vi "source sim.vi"() -> ()   [LabVIEW 2016]
uses:
  <vilib>/Platform/TimedLoop/XDataNode/timing_clust.ctl
  <vilib>/Platform/TimedLoop/XDataNode/nitl_modes.ctl
  <vilib>/Platform/TimedLoop/XDataNode/wakeup.ctl
  <vilib>/Analysis/baseanly.llb/Mean (CDB).vi
  <vilib>/platform/TimedLoop/XDataNode/XDataNode.xnode
  <vilib>/Platform/TimedLoop/XDataNode/XDNodeRunTimeDep.lvlib
  <vilib>/Analysis/NI_AALBase.lvlib
panel:
  in  "Rotate CCW":bool
  in  "Rotate CW":bool
  in  "Stop Button":bool
  out "Simulation Time (Seconds)":dbl=0.12610000000000002 format="%_4g"
  out "Frequency (Hz)":dbl=34.3
  out "Wavenumber (Radians / Meter)":dbl=0.6283185307179586
  in  "Delete Source":bool
  in  "Add Source":bool
  in  "Velocity of Propogation (m/s)":dbl=343.0 min=200.0 max=400.0 step=1.0
  in  "dT":dbl=0.0001
  in  "Spatial Resolution (meters)":dbl=0.25 min=0.1 max=10.0 step=0.1
  in  "Extent (Meters)":dbl=50.0 min=50.0 max=400.0 step=1.0
  in  "Wavelength (meters)":dbl=10.0
  out "Intensity Graph":dbl[][](graph)
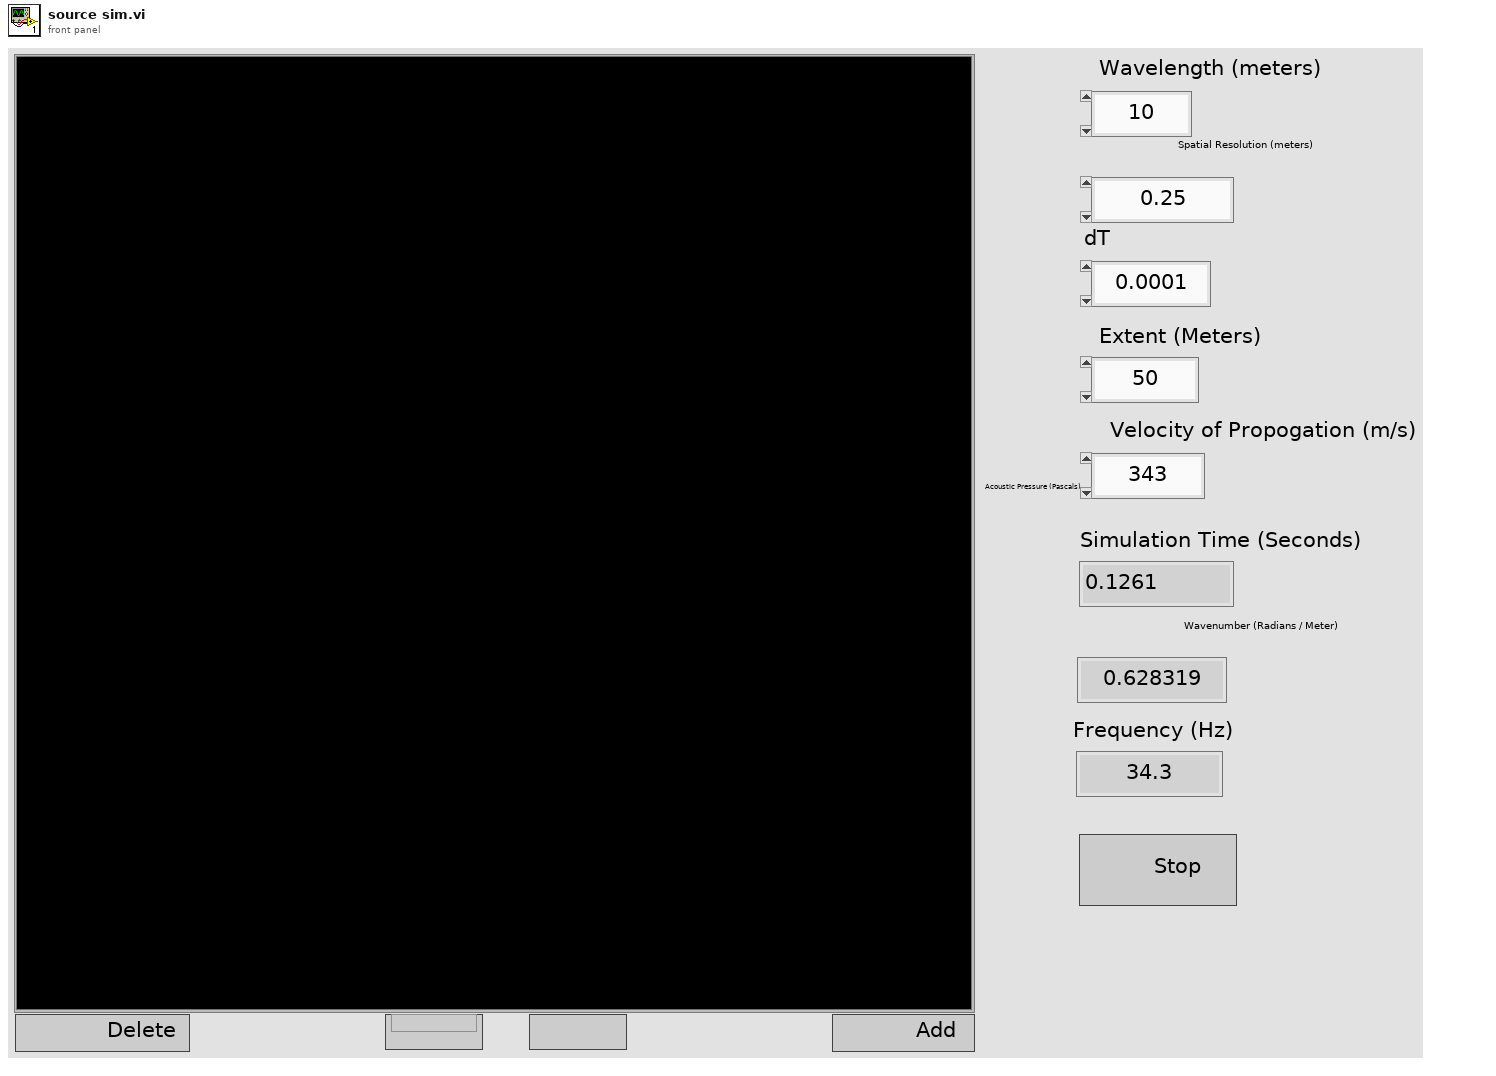
[diagram p1: front panel]
types:
  T1 = typedef "XDNodeRunTimeDep.lvlib/timing_clust.ctl" = cluster{"Expected End [f-1]":u64, "Actual End [f-1]":u64, "Finished Late? [f-1]":bool, "Expected End [i-1]":u64, "Actual End [i-1]":u64, "Finished Late? [i-1]":bool, "Expected Start [i]":u64, "Actual Start [i]":u64, "Expected Start [f]":u64, "Actual Start [f]":u64, "Source Name":string, "Structure Name":string, "Period":i64, "Deadline":i64, "Offset":i64, "Start":i64, "Priority":i32, "Timeout":i32, "Mode":T2, "Wakeup Reason":T3, "Error":errorcluster, "Source Type":string, "Secondary Source Type":string, "Global End Time":u64, "Global Start Time":u64, "Frame Duration":u64, "Iteration Duration":u64, "Assigned CPU":i32, "I/O Scan Engine Mode":u32}
  T2 = typedef "XDNodeRunTimeDep.lvlib/nitl_modes.ctl" = enum32{"No Change", "Process missed periods, maintain original phase", "Discard missed periods, maintain original phase", "Process missed periods, ignore original phase", "Discard missed periods, ignore original phase"}
  T3 = typedef "XDNodeRunTimeDep.lvlib/wakeup.ctl" = enum32{"Normal", "Aborted", "Asynchronous wakeup", "Timing source error", "Timed loop error", "Timeout"}
  T4 = cluster{"Name":string, "Color":u32, "Style":u8, "Point Style":u8, "Name Visible":bool, "Allow Drag":bool, "Cursor Mode":u32, "Plot":i32, "Index":i32, "Position":cluster{"X":dbl, "Y":dbl}, "X Scale":u32, "Y Scale":u32, "Watch Plots":i32[], "Watch All Plots":bool, "Plot Area":i32, "Label Offset":cluster{"X":dbl, "Y":dbl}}
  T5 = typedef "LVCursorListTypeDef.ctl" = cluster{"Name":string, "Color":u32, "Style":u8, "Point Style":u8, "Name Visible":bool, "Allow Drag":bool, "Cursor Mode":u32, "Plot":i32, "Index":i32, "Position":cluster{"X":dbl, "Y":dbl}, "X Scale":u32, "Y Scale":u32, "Watch Plots":i32[], "Watch All Plots":bool, "Plot Area":i32, "Label Offset":cluster{"X":dbl, "Y":dbl}}[]
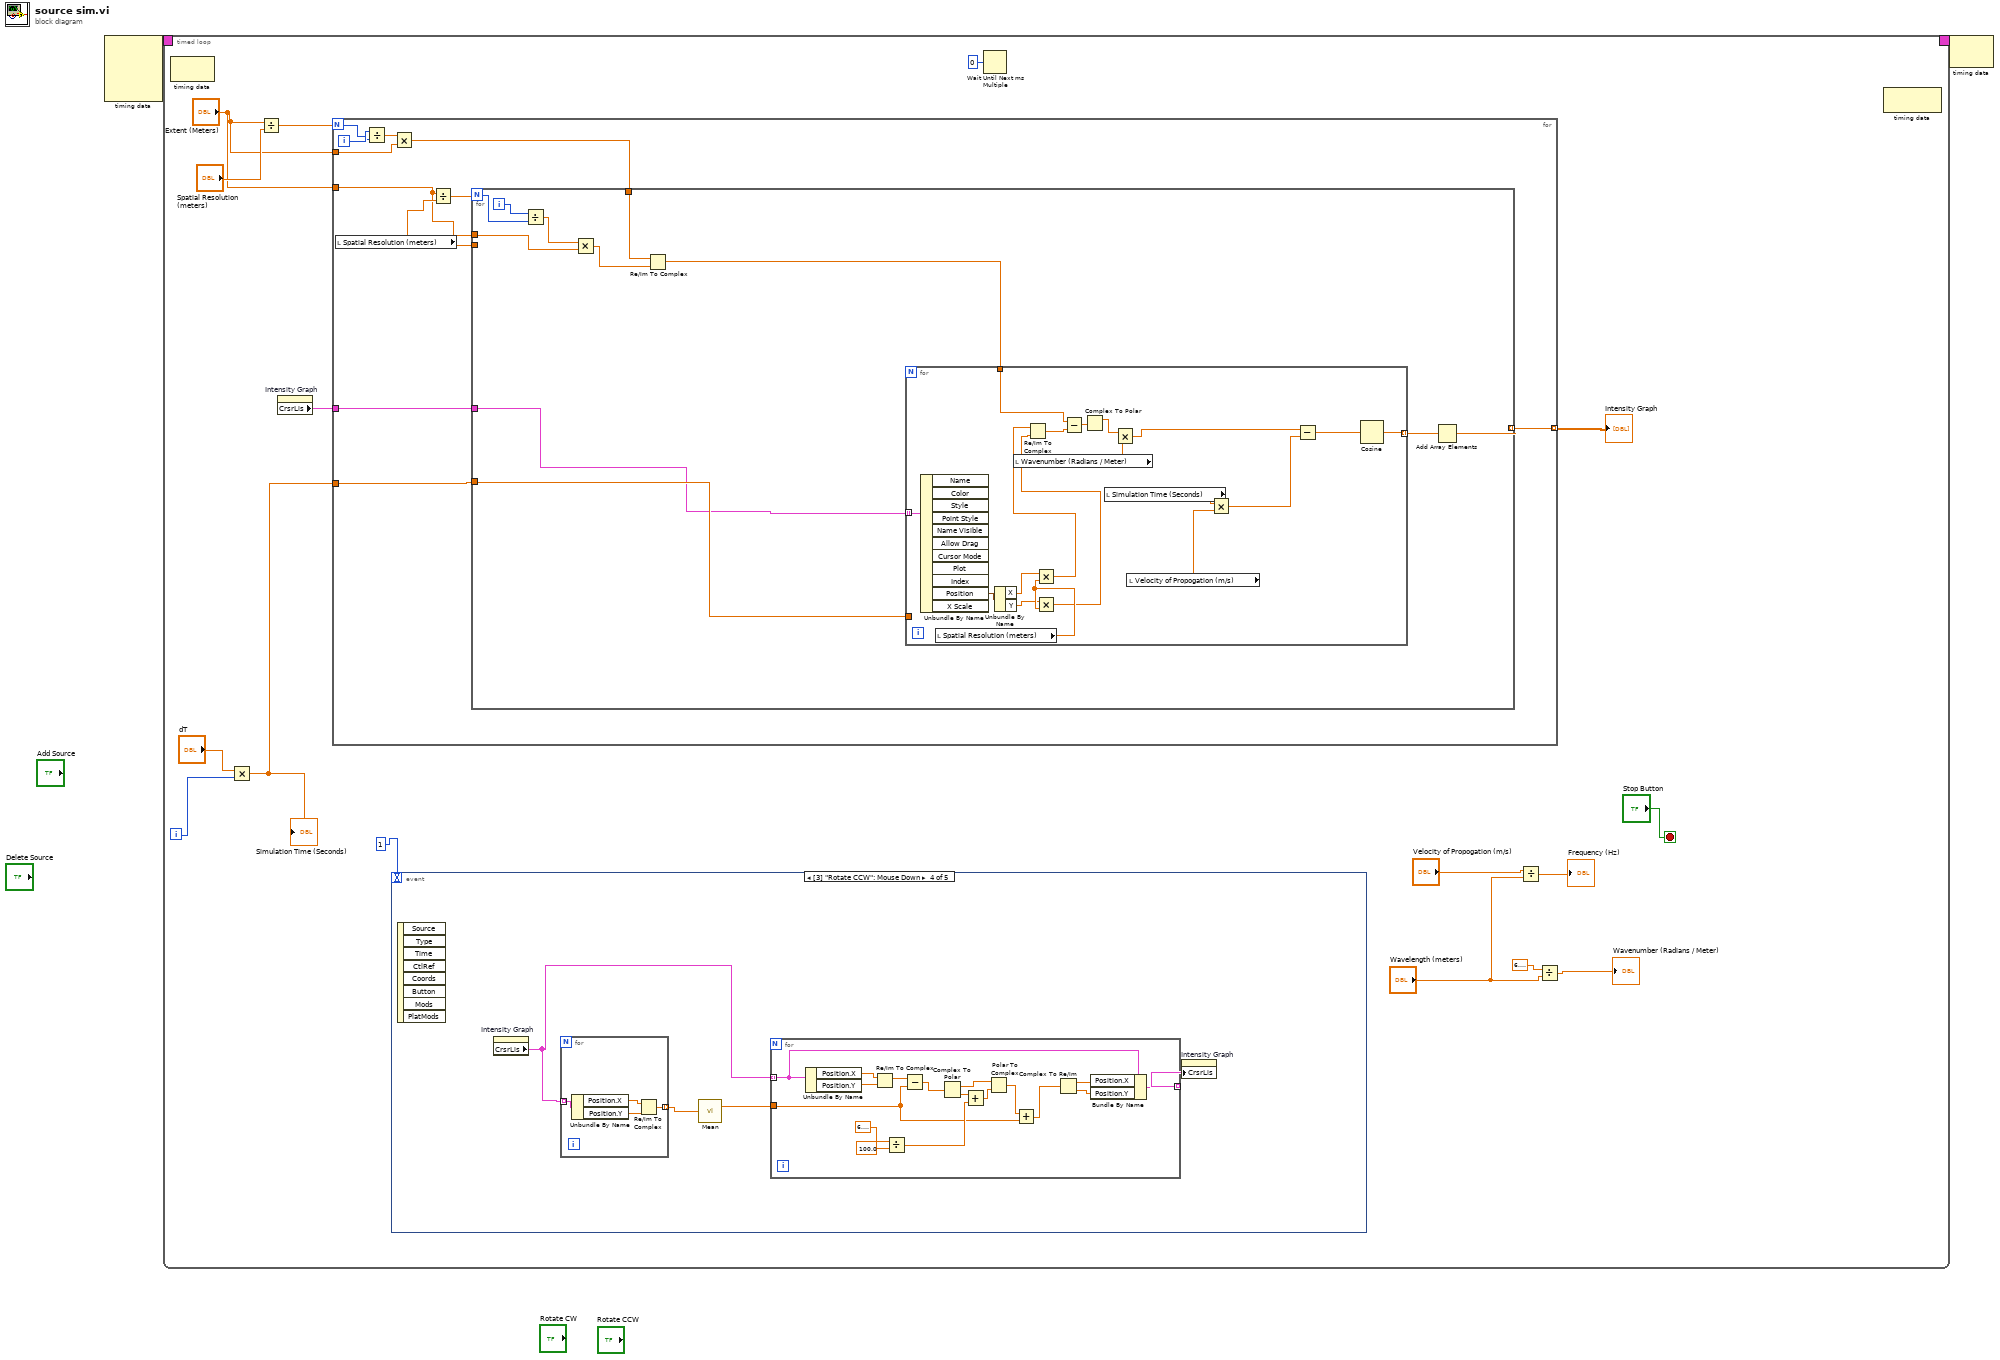
[diagram p0: block diagram]
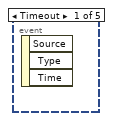
[diagram p2: hidden frame]
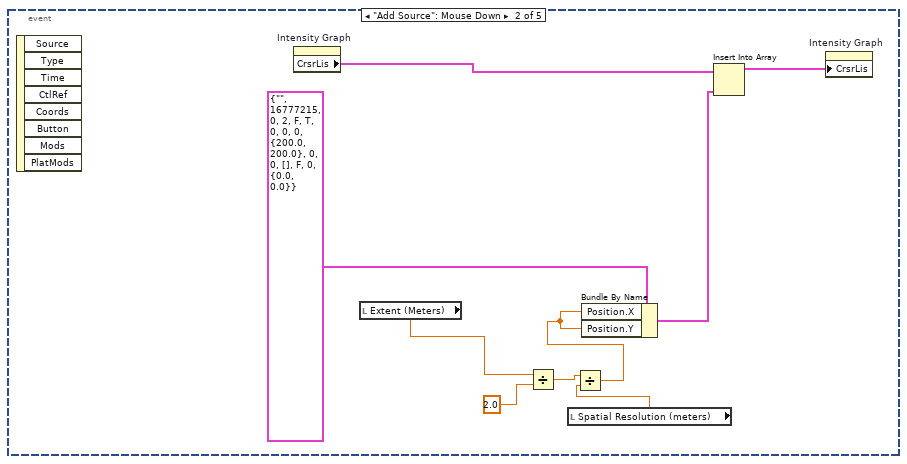
[diagram p3: hidden frame]
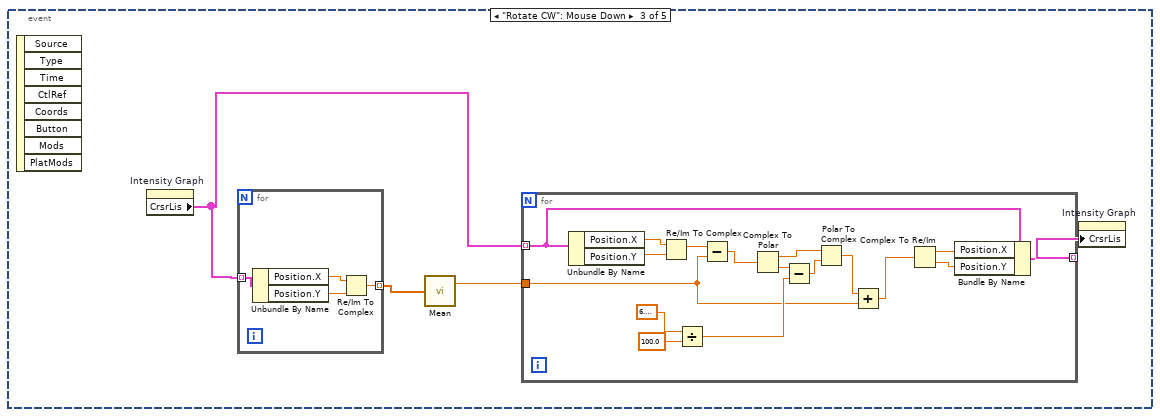
[diagram p4: hidden frame]
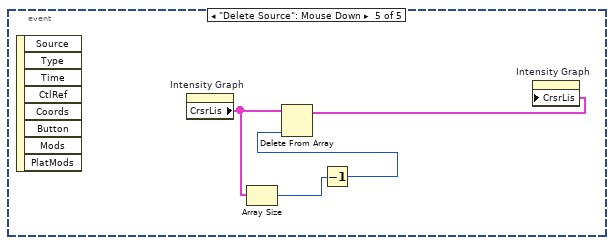
[diagram p5: hidden frame]
diagram:
  n1 = node-c288() -> (w2:T1)  [unwired: 4 in]
  n2 = timed-loop {
    timing: w2 -> [_]
    timing-out: [_] -> w1
    i -> [w13]
    stop <- "Stop Button" stop-if-true
    n3 = node-c288() -> ()  [unwired: 1 in, 1 out]
    n4 = Multiply(x="dT", y=w13) -> (x*y=w16:dbl)
    "Simulation Time (Seconds)" <- w16
    n5 = Divide(x="Extent (Meters)", y="Spatial Resolution (meters)") -> (x/y=w18:dbl)
    n6 = property on="Intensity Graph" class="IntGraph (strict)"() -> ("CrsrLis"=w12:T5)  [unwired: 2 in, 2 out]
    n7 = for {
      N: w18 -> [w90]
      tunnel: "Extent (Meters)" -> [w93]
      tunnel: w16 -> [w88]
      tunnel: w12 -> [w86]
      tunnel: "Extent (Meters)" -> [w85]
      tunnel: [w84] -> w9 mode=indexing
      i -> [w91]
      n8 = local read "Spatial Resolution (meters)"() -> (w92:dbl)
      n9 = Divide(x=w91, y=w90) -> (x/y=w94:dbl)
      n10 = Multiply(x=w94, y=w93) -> (x*y=w89:dbl)
      n11 = Divide(x=w85, y=w92) -> (x/y=w87:dbl)
      n12 = for {
        N: w87 -> [w104]
        tunnel: w92 -> [_]
        tunnel: w89 -> [w103]
        tunnel: w88 -> [w98]
        tunnel: w85 -> [w101]
        tunnel: w86 -> [w97]
        tunnel: [w95] -> w84 mode=indexing
        i -> [w105]
        n13 = Divide(x=w105, y=w104) -> (x/y=w102:dbl)
        n14 = Multiply(x=w102, y=w101) -> (x*y=w100:dbl)
        n15 = Re/Im To Complex(1:w100, 2:w103) -> (0:w99:cdb)
        n16 = for {
          tunnel: w97 -> [w123] mode=indexing
          tunnel: w99 -> [w119]
          tunnel: [w118] -> w96 mode=indexing
          tunnel: w98 -> [_]
          n17 = Unbundle By Name(w123) -> ("Position"=w114:cluster{"X":dbl, "Y":dbl})  [unwired: 10 out]
          n18 = local read "Spatial Resolution (meters)"() -> (w115:dbl)
          n19 = Unbundle By Name(w114) -> ("X"=w113:dbl, "Y"=w112:dbl)
          n20 = local read "Wavenumber (Radians / Meter)"() -> (w108:dbl)
          n21 = Multiply(x=w113, y=w115) -> (x*y=w110:dbl)
          n22 = Multiply(x=w112, y=w115) -> (x*y=w109:dbl)
          n23 = Re/Im To Complex(1:w109, 2:w110) -> (0:w116:cdb)
          n24 = Subtract(x=w119, y=w116) -> (x-y=w120:cdb)
          n25 = Complex To Polar(r * e^(i*theta)=w120) -> (r=w117:dbl)  [unwired: 1 out]
          n26 = local read "Simulation Time (Seconds)"() -> (w106:dbl)
          n27 = Multiply(x=w117, y=w108) -> (x*y=w122:dbl)
          n28 = local read "Velocity of Propogation (m/s)"() -> (w107:dbl)
          n29 = Multiply(x=w106, y=w107) -> (x*y=w121:dbl)
          n30 = Subtract(x=w122, y=w121) -> (x-y=w111:dbl)
          n31 = Cosine(x=w111) -> (cos(x)=w118:dbl)
        }
        n32 = Add Array Elements(numeric array=w96) -> (sum=w95:dbl)
      }
    }
    "Intensity Graph" <- w9
    n33 = event shown="[3] \"Rotate CCW\": Mouse Down" {
      selector: _ -> [_ _ _ _ _]
      dyn-events: _ -> [_ _ _ _ _]
      timeout: 1 -> [_ _ _ _ _]
      event Timeout {
        n34 = event-data() -> ()  [unwired: 1 in, 3 out]
      }
      event "Add Source": Mouse Down {
        n35 = event-data() -> ()  [unwired: 1 in, 8 out]
        n36 = property on="Intensity Graph" class="IntGraph (strict)"() -> ("CrsrLis"=w23:T5)  [unwired: 2 in, 2 out]
        n37 = local read "Extent (Meters)"() -> (w22:dbl)
        n38 = Divide(x=w22, y=2.0) -> (x/y=w21:dbl)
        n39 = local read "Spatial Resolution (meters)"() -> (w20:dbl)
        n40 = Divide(x=w21, y=w20) -> (x/y=w19:dbl)
        n41 = Bundle By Name(cluster=T4 {"Name"="", "Color"=16777215, "Style"=0, "Point Style"=2, "Name Visible"=FALSE, "Allow Drag"=TRUE, "Cursor Mode"=0, "Plot"=0, "Index"=0, "Position"={"X"=200.0, "Y"=200.0}, "X Scale"=0, "Y Scale"=0, "Watch Plots"=[], "Watch All Plots"=FALSE, "Plot Area"=0, "Label Offset"={"X"=0.0, "Y"=0.0}} ("new element/subarray"), "Position.X"=w19, "Position.Y"=w19) -> (w24:T4)
        n42 = Insert Into Array(array=w23, new element=w24) -> (w27:T5)  [unwired: 1 in]
        n43 = property on="Intensity Graph" class="IntGraph (strict)"("CrsrLis"=w27) -> ()  [unwired: 2 in, 2 out]
      }
      event "Rotate CW": Mouse Down {
        n44 = event-data() -> ()  [unwired: 1 in, 8 out]
        n45 = property on="Intensity Graph" class="IntGraph (strict)"() -> ("CrsrLis"=w31:T5)  [unwired: 2 in, 2 out]
        n46 = for {
          tunnel: w31 -> [w52] mode=indexing
          tunnel: [w49] -> w29 mode=indexing
          n47 = Unbundle By Name(w52) -> ("Position.X"=w50:dbl, "Position.Y"=w51:dbl)
          n48 = Re/Im To Complex(1:w51, 2:w50) -> (0:w49:cdb)
        }
        n49 = call-poly <vilib>:"Mean.vi"("X"=w29) -> ("mean"=w28:cdb)  [unwired: 1 out]
        n50 = for {
          tunnel: w31 -> [w38] mode=indexing
          tunnel: [w37] -> w30 mode=indexing
          tunnel: w28 -> [w35]
          n51 = Unbundle By Name(w38) -> ("Position.X"=w48:dbl, "Position.Y"=w47:dbl)
          n52 = Re/Im To Complex(1:w47, 2:w48) -> (0:w46:cdb)
          n53 = Divide(x=6.283185307179586, y=100.0) -> (x/y=w41:dbl)
          n54 = Subtract(x=w46, y=w35) -> (x-y=w45:cdb)
          n55 = Complex To Polar(r * e^(i*theta)=w45) -> (r=w39:dbl, theta=w44:dbl)
          n56 = Subtract(x=w44, y=w41) -> (x-y=w40:dbl)
          n57 = Polar To Complex(1:w40, 2:w39) -> (0:w36:cdb)
          n58 = Add(x=w36, y=w35) -> (x+y=w32:cdb)
          n59 = Complex To Re/Im(x + iy=w32) -> (x=w34:dbl, y=w33:dbl)
          n60 = Bundle By Name(cluster=w38, "Position.X"=w34, "Position.Y"=w33) -> (w37:T4)
        }
        n61 = property on="Intensity Graph" class="IntGraph (strict)"("CrsrLis"=w30) -> ()  [unwired: 2 in, 2 out]
      }
      event "Rotate CCW": Mouse Down {
        n62 = event-data() -> ()  [unwired: 1 in, 8 out]
        n63 = property on="Intensity Graph" class="IntGraph (strict)"() -> ("CrsrLis"=w56:T5)  [unwired: 2 in, 2 out]
        n64 = for {
          tunnel: w56 -> [w77] mode=indexing
          tunnel: [w74] -> w54 mode=indexing
          n65 = Unbundle By Name(w77) -> ("Position.X"=w75:dbl, "Position.Y"=w76:dbl)
          n66 = Re/Im To Complex(1:w76, 2:w75) -> (0:w74:cdb)
        }
        n67 = call-poly <vilib>:"Mean.vi"("X"=w54) -> ("mean"=w53:cdb)  [unwired: 1 out]
        n68 = for {
          tunnel: w56 -> [w63] mode=indexing
          tunnel: [w62] -> w55 mode=indexing
          tunnel: w53 -> [w60]
          n69 = Unbundle By Name(w63) -> ("Position.X"=w73:dbl, "Position.Y"=w72:dbl)
          n70 = Re/Im To Complex(1:w72, 2:w73) -> (0:w71:cdb)
          n71 = Divide(x=6.283185307179586, y=100.0) -> (x/y=w66:dbl)
          n72 = Subtract(x=w71, y=w60) -> (x-y=w70:cdb)
          n73 = Complex To Polar(r * e^(i*theta)=w70) -> (r=w64:dbl, theta=w69:dbl)
          n74 = Add(x=w69, y=w66) -> (x+y=w65:dbl)
          n75 = Polar To Complex(1:w65, 2:w64) -> (0:w61:cdb)
          n76 = Add(x=w61, y=w60) -> (x+y=w57:cdb)
          n77 = Complex To Re/Im(x + iy=w57) -> (x=w59:dbl, y=w58:dbl)
          n78 = Bundle By Name(cluster=w63, "Position.X"=w59, "Position.Y"=w58) -> (w62:T4)
        }
        n79 = property on="Intensity Graph" class="IntGraph (strict)"("CrsrLis"=w55) -> ()  [unwired: 2 in, 2 out]
      }
      event "Delete Source": Mouse Down {
        n80 = event-data() -> ()  [unwired: 1 in, 8 out]
        n81 = property on="Intensity Graph" class="IntGraph (strict)"() -> ("CrsrLis"=w81:T5)  [unwired: 2 in, 2 out]
        n82 = Array Size(array=w81) -> (size(s)=w80:i32)
        n83 = Decrement(x=w80) -> (x-1=w78:i32)
        n84 = Delete From Array(array=w81, index=w78) -> (array with subset deleted=w79:T5)  [unwired: 1 in, 1 out]
        n85 = property on="Intensity Graph" class="IntGraph (strict)"("CrsrLis"=w79) -> ()  [unwired: 2 in, 2 out]
      }
    }
    n86 = Wait Until Next ms Multiple(millisecond multiple=u32 0) -> ()  [unwired: 1 out]
    n87 = Divide(x="Velocity of Propogation (m/s)", y="Wavelength (meters)") -> (x/y=→"Frequency (Hz)":dbl)
    n88 = Divide(x=6.283185307179586, y="Wavelength (meters)") -> (x/y=→"Wavenumber (Radians / Meter)":dbl)
    n89 = node-c288() -> ()  [unwired: 1 in, 1 out]
  }
  n90 = node-c288(w1) -> ()  [unwired: 1 out]
